vi "Filter Control Drop Event.vi"(8 "error in (no error)":errorcluster, 10 "ControlDropMsg":refnum<class "ControlDropMsg.lvclass">, 11 "IEventFilter in":refnum<class "IEventFilter.lvclass">) -> (0 "error out":errorcluster, 1 "Discard?":bool, 3 "IEventFilter out":refnum<class "IEventFilter.lvclass">)   [LabVIEW 2015, in "ActorEvents.lvlib" / "IEventFilter.lvclass"]
uses:
  IEventFilter.lvclass
  IEventAggregator Messages/ControlDropMsg/ControlDropMsg.lvclass
panel:
  # "No additional\nEvent Data"
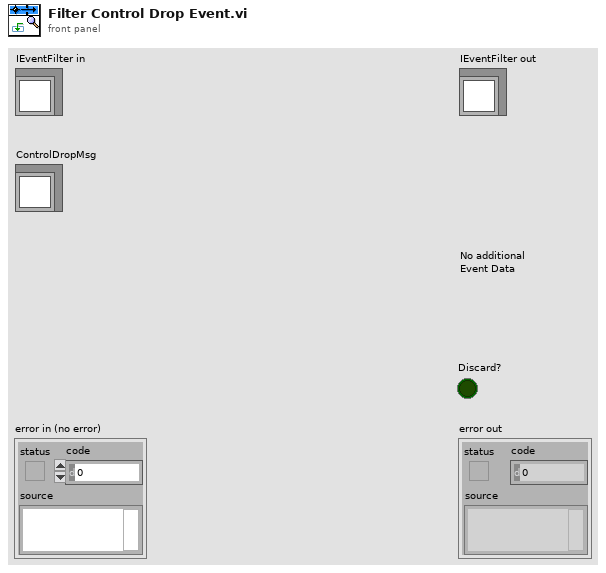
[diagram p1: front panel]
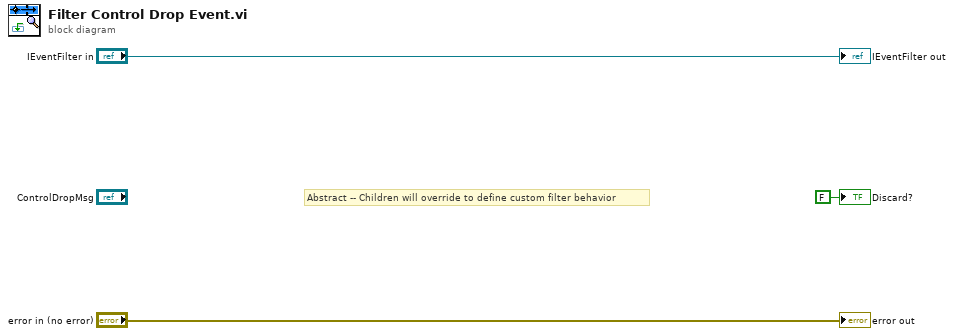
[diagram p0: block diagram]
diagram:
  # "Abstract -- Children will override to define custom filter behavior"
  "error out" <- "error in (no error)"
  "IEventFilter out" <- "IEventFilter in"
  "Discard?" <- FALSE ("Discard?")
